vi "Read Header.vi"(0 "TIFF Data in":u8[](array[numeric])) -> (1 "TIFF Data out":u8[](array[numeric]), 2 "Litt/BigEnd":bool, 3 "ImFileDirectOffs":u32, 4 "IsTIFF?":bool)   [LabVIEW 2015, in "Tiff reader.lvlib"]
doc: "Reads the header of a tiff file to determine the version number and the location of the image data in the file. Format determines whether the image file is coded LSB or MSB, although the rest of the routines only understand PC image data !"
uses:
  Tiff reader.lvlib
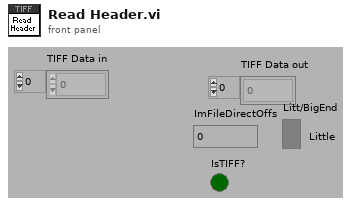
[diagram p1: front panel]
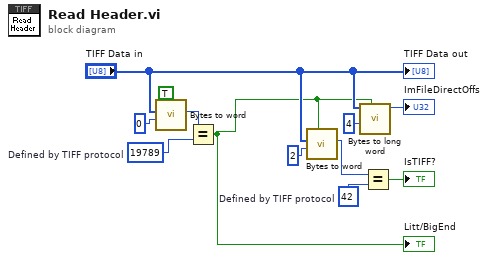
[diagram p0: block diagram]
diagram:
  w3 = u16 42  # Defined by TIFF protocol
  w9 = u16 19789  # Defined by TIFF protocol
  n1 = call "Bytes to word.vi"("Litt/BigEnd"=TRUE, "Index"=0, "Image Data in"="TIFF Data in") -> ("Word"=w8:u16)  [unwired: 1 in, 5 out]
  n2 = Equal?(x=w8, y=w9) -> (x = y?=w11:bool)
  "Litt/BigEnd" <- w11
  n3 = call "Bytes to word.vi"("Litt/BigEnd"=w11, "Index"=2, "Image Data in"="TIFF Data in") -> ("Word"=w1:u16)  [unwired: 1 in, 5 out]
  n4 = call "Bytes to long word.vi"("Litt/BigEnd"=w11, "Index"=4, "Image Data in"="TIFF Data in") -> ("U32"=→"ImFileDirectOffs":u32)  [unwired: 6 out]
  n5 = Equal?(x=w1, y=w3) -> (x = y?=→"IsTIFF?":bool)
  "TIFF Data out" <- "TIFF Data in"
